vi "TCP Data Stream.vi"(0 "Address":string, 1 "Port":u16, 2 "Data IN":dbl[][](array[numeric]), 3 "String IN":string, 5 "Error IN":errorcluster, 6 "Mode":T1, 9 "Write String (F)":bool, 11 "TCP Stream Ref":refnum<vi>) -> (14 "Data OUT":dbl[][](array[numeric]), 15 "New Data?":bool, 16 "Connected?":bool, 17 "String OUT":string, 19 "Error OUT":errorcluster)   [LabVIEW 2019]
uses:
  Type Defs and Controls/TCP Data Stream Mode.ctl
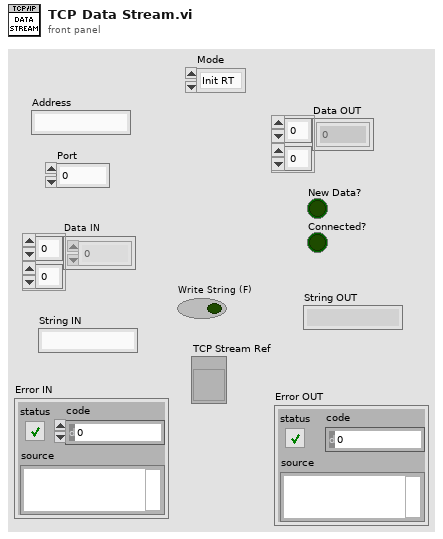
[diagram p1: front panel]
types:
  T1 = typedef "TCP Data Stream Mode.ctl" = enum16{"Init RT", "Init PC", "Connect RT", "Connect PC", "Write Data", "Read Data", "Close"}
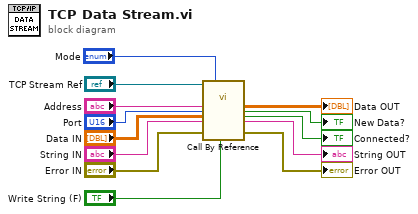
[diagram p0: block diagram]
diagram:
  n1 = call-by-ref "?"(reference="TCP Stream Ref", "Address"="Address", "Port"="Port", "Data IN"="Data IN", "String IN"="String IN", "Error IN"="Error IN", "Mode"="Mode", "Write String (F)"="Write String (F)") -> ("Data OUT"=→"Data OUT":dbl[][], "New Data?"=→"New Data?":bool, "Connected?"=→"Connected?":bool, "String OUT"=→"String OUT":string, "Error OUT"=→"Error OUT":errorcluster)  [unwired: 9 in, 2 out]
